vi "DSF.Engine.Framework.Rx.Inline.Start.vi"(8 "error in (no error)":errorcluster, 11 "Framework in":refnum<class "DSF.Engine.Framework.lvclass">) -> (0 "error out":errorcluster, 3 "Framework out":refnum<class "DSF.Engine.Framework.lvclass">)   [LabVIEW 2017, in "DSF.Engine.lvlib" / "DSF.Engine.Framework.lvclass"]
uses:
  DSF.Engine.Framework.lvclass
  DSF.Engine.Framework.lvclass/DSF.Engine.Framework.ctl
  Plugin/DSF.Engine.Plugin.lvclass/DSF.Engine.Plugin.ctl
  Timing/DSF.Engine.Timing.lvclass/DSF.Engine.Timing.ctl
  Transfer/DSF.Engine.Transfer Group.lvclass/DSF.Engine.Transfer Group.ctl
  Thread Pool/DSF.Engine.Pool.lvclass/DSF.Engine.Pool.ctl
  Transceiver/DSF.Engine.Transceiver Thread.lvclass/DSF.Engine.Transceiver Thread.ctl
  Interface/DSF.Engine.Interface.lvclass/DSF.Engine.Interface.ctl
  Plugin/DSF.Engine.Plugin.Get Inline Rx Transfer Groups.vi
  Plugin/DSF.Engine.Plugin.Set Inline Rx Transfer Groups.vi
  Plugin/DSF.Engine.Plugin.Rx.Transfer Group.Send.vi
  Plugin/DSF.Engine.Plugin.Transfer Group.Iteration.Increment.vi
  Plugin/DSF.Engine.Plugin.Get Timing.vi
  Timing/DSF.Engine.Timing.Is Active Cycle.vi
  Plugin/DSF.Engine.Plugin.Transceiver Thread.Obtain.vi
  Transceiver/DSF.Engine.Transceiver Thread.Command.Transfer Group.vi
  Transfer/DSF.Engine.Transfer Group.Increment Iteration.vi
  Timing/DSF.Engine.Timing.Get Decimation.vi
  Timing/DSF.Engine.Timing.Get Offset.vi
  Thread Pool/DSF.Engine.Pool.ID.Obtain ID from Pool.vi
  Plugin/DSF.Engine.Plugin.Get Thread ID Pool.vi
  Plugin/DSF.Engine.Plugin.Get Transceiver Thread.vi
  Transceiver/DSF.Engine.Transceiver Thread.Get Interface.vi
  Interface/DSF.Engine.Interface.Transceiver.Write.vi
  Interface/DSF.Engine.Interface.Transceiver.Write.Command.vi
  Transfer/DSF.Engine.Transfer Group.Get ID.vi
  Timing/DSF.Engine.Timing.Get Iteration.vi
  Transfer/DSF.Engine.Transfer Group.Get Timing.vi
  Transfer/DSF.Engine.Transfer Group.Set Timing.vi
  Timing/DSF.Engine.Timing.Iteration.Increment.vi
  Thread Pool/DSF.Engine.Pool.Read FIFO.vi
  Interface/DSF.Engine.Interface.RT FIFO.Write.16B.vi
  Interface/DSF.Engine.Interface.Get Command FIFO.vi
  Timing/DSF.Engine.Timing.Set Iteration.vi
  Thread Pool/DSF.Engine.Pool.Get FIFO.vi
  Thread Pool/DSF.Engine.Pool.ID.lvclass
  C:/Git/DSF/Source/Engine/Classes/Thread Pool/DSF.Engine.Pool.lvclass
  Interface/DSF.Engine.Interface.Transceiver.lvclass
  C:/Git/DSF/Source/Engine/Classes/Interface/DSF.Engine.Interface.lvclass
  Transceiver/DSF.Engine.Transceiver Thread.lvclass
  Plugin/DSF.Engine.Plugin.lvclass
  State/Framework State.lvclass
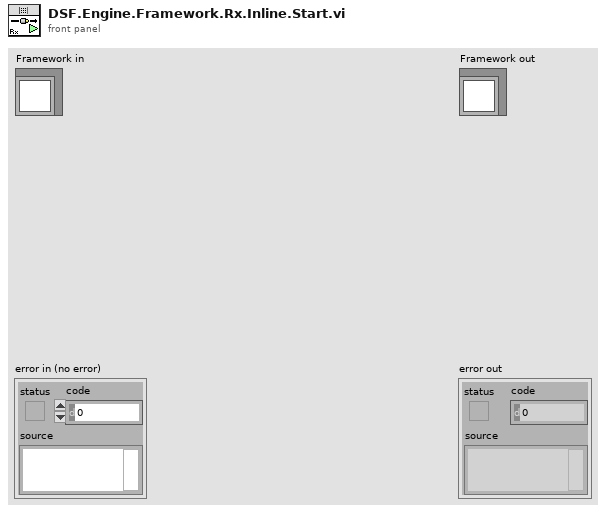
[diagram p1: front panel]
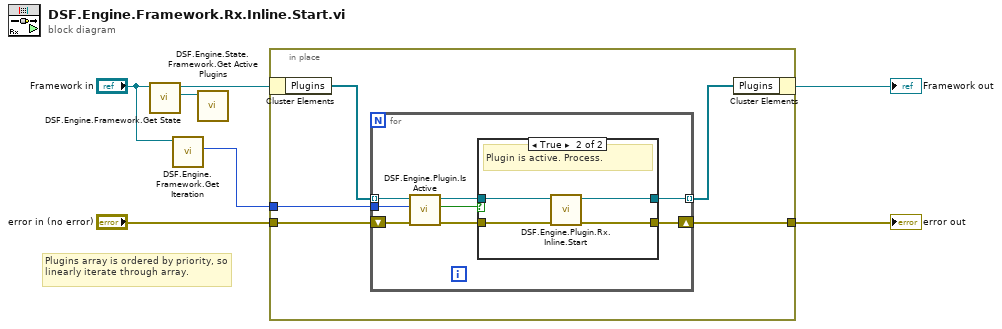
[diagram p0: block diagram]
diagram:
  # "Plugins array is ordered by priority, so linearly iterate through array."
  n1 = call "DSF.Engine.Framework.Get State.vi"("Framework in"="Framework in") -> ("State"=w5:refnum<class "Framework State.lvclass">, "Framework out"=w1:refnum<class "DSF.Engine.Framework.lvclass">)  [unwired: 9 in]
  n2 = call "DSF.Engine.Framework.Get Iteration.vi"("Framework in"="Framework in") -> ("iteration"=w4:u64)  [unwired: 9 in, 1 out]
  n3 = call "DSF.Engine.State.Framework.Get Active Plugins.vi"("Framework State in"=w5) -> ()  [unwired: 9 in, 2 out]
  n4 = in-place {
    in-place-border: "error in (no error)" -> [w12]
    in-place-border: [w11] -> w6
    in-place-border: w4 -> [w10]
    n5 = in-place-cluster #1(w1) -> ("Plugins"=w9:refnum<class "DSF.Engine.Plugin.lvclass">[])
    n6 = for {
      tunnel: w9 -> [w13] mode=indexing
      tunnel: [w19] -> w8 mode=indexing
      shift-right: [w18] -> w11
      shift-left: w12 -> [w17]
      tunnel: w10 -> [w15]
      n7 = call "DSF.Engine.Plugin.Is Active.vi"("cycle count"=w15, "Plugin in"=w13) -> ("active this cycle?"=w14:bool, "Plugin out"=w16:refnum<class "DSF.Engine.Plugin.lvclass">)  [unwired: 8 in]
      n8 = case shown="True" w14 {
        tunnel: w16 -> [w21 w25]
        tunnel: [w21 w24] -> w19
        tunnel: [w20 w22] -> w18
        tunnel: w17 -> [w20 w23]
        frame False {
          # "Plugin is not active. Skip."
        }
        frame True {
          # "Plugin is active. Process."
          n9 = call "DSF.Engine.Plugin.Rx.Inline.Start.vi"("error in (no error)"=w23, "Plugin in"=w25) -> ("error out"=w22:errorcluster, "Plugin out"=w24:refnum<class "DSF.Engine.Plugin.lvclass">)  [unwired: 8 in]
        }
      }
    }
    n10 = in-place-cluster #1("Plugins"=w8) -> (→"Framework out":refnum<class "DSF.Engine.Framework.lvclass">)
  }
  "error out" <- w6
